vi "Write Results.vi"(8 "error in":errorcluster, 11 "Peer Review in":refnum<class "Peer Review.lvclass">) -> (0 "error out":errorcluster, 3 "Peer Review out":refnum<class "Peer Review.lvclass">)   [LabVIEW 2020, in "Peer Review.lvclass"]
uses:
  Peer Review.lvclass
  Peer Review.lvclass/Peer Review.ctl
  TypeDefs/File Info.ctl
  TypeDefs/File State.ctl
  TypeDefs/VI Type.ctl
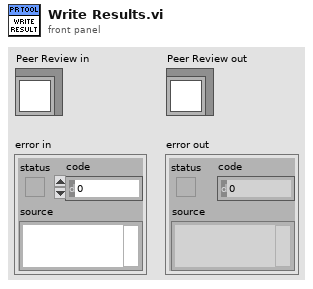
[diagram p1: front panel]
types:
  T1 = typedef "Peer Review.lvclass/File Info.ctl" = cluster{"File ID":i32, "Commit ID":i32, "Reviewed Hash":string, "Relative Path":string, "File Path":path, "File Checksum":string, "State":T2, "FP Changes":i32, "BD Changes":i32, "FP Bounds Error":dbl, "BD Bounds Error":dbl, "Lines Added":i32, "Lines Removed":i32, "Analysis Passes":i32, "Analysis Fails":i32, "Attribute Changes":i32, "Reentrancy Changes":string, "Cyclomatic Complexity":i32, "Node Count":i32, "Revision Number":u32, "LabVIEW Version":string, "Description":string, "Master Path":path, "Master Checksum":string, "VI Type":T3, "LabVIEW File":bool, "Review Complete":bool, "File Ref":refnum<vi>}
  T2 = typedef "Peer Review.lvclass/File State.ctl" = enum16{"Interrogation Needed", "Modified", "Deleted", "Added", "Matches Previous", "No Changes", "Moved"}
  T3 = typedef "Peer Review.lvclass/VI Type.ctl" = enum32{"invalid VI type", "Standard VI", "Control VI", "Global VI", "Polymorphic VI", "Configuration VI", "SubSystem", "Facade VI", "Method VI", "Statechart Diagram VI"}
  T4 = enum16{"open", "replace", "create", "open or create", "replace or create", "replace or create with confirmation"}
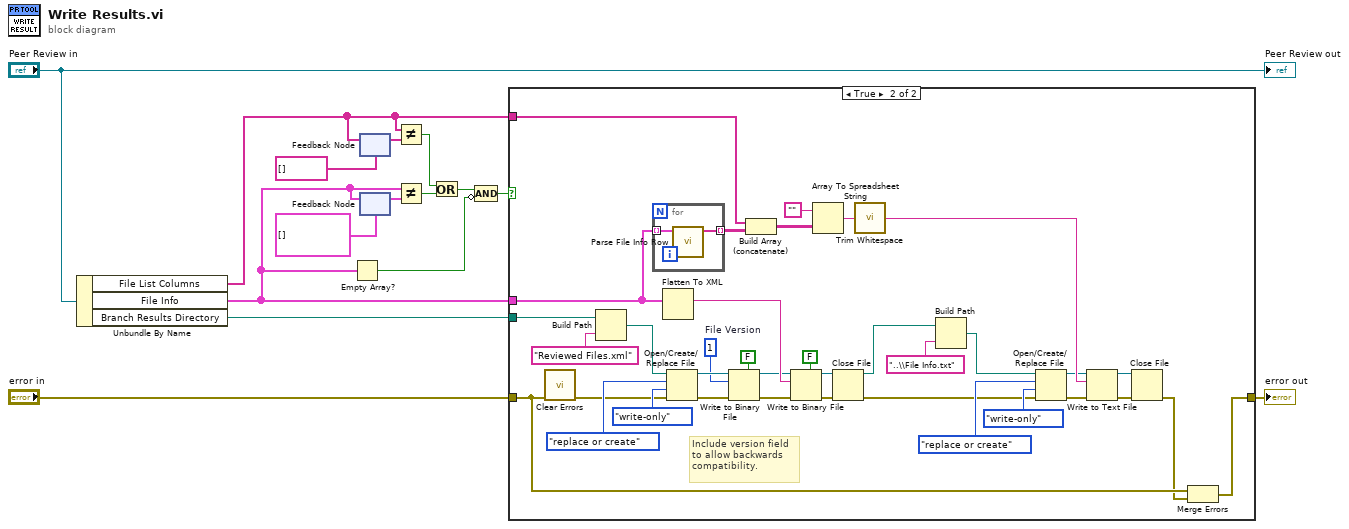
[diagram p0: block diagram]
diagram:
  n1 = Unbundle By Name("Peer Review in") -> ("File List Columns"=w2:string[], "File Info"=w1:T1[], "Branch Results Directory"=w14:path)
  n2 = Empty Array?(array=w1) -> (empty?=w4:bool)
  n3 = feedback #1(string[] [] ("File List Columns")) -> (w10:string[])
  n4 = feedback-in #1(w2) -> ()
  n5 = feedback-in #2(w1) -> ()
  n6 = feedback #2(T1[] [] ("File Info")) -> (w11:T1[])
  n7 = Not Equal?(x=w2, y=w10) -> (x != y?=w9:bool)
  n8 = Not Equal?(x=w1, y=w11) -> (x != y?=w8:bool)
  n9 = Or(x=w9, y=w8) -> (x .or. y?=w5:bool)
  n10 = Compound Arithmetic op=AND(w5, invert w4) -> (w3:bool)
  n11 = case shown="True" w3 {
    tunnel: [w16 w17] -> w12
    tunnel: w14 -> [_ w45]
    tunnel: w1 -> [_ w52]
    tunnel: w2 -> [_ w50]
    tunnel: "error in" -> [w16 w19]
    frame False {
      # "No results to write (or unchanged), so do nothing."
    }
    frame True {
      w33 = u32 1  # File Version
      # "Include version field\nto allow backwards\ncompatibility."
      n12 = call <vilib>:"Clear Errors.vi"("error in (no error)"=w19) -> ("error out"=w20:errorcluster)  [unwired: 5 in, 1 out]
      n13 = Build Path(base path=w45, name or relative path="Reviewed Files.xml") -> (appended path=w39:path)
      n14 = for {
        tunnel: w52 -> [w54] mode=indexing
        tunnel: [w53] -> w51 mode=indexing
        n15 = call "Parse File Info Row.vi"("File Info"=w54) -> ("Column Fields"=w53:string[])  [unwired: 10 in]
      }
      n16 = Flatten To XML(6:w52) -> (2:w38:string)
      n17 = Open/Create/Replace File(file path (use dialog)=w39, error in=w20, operation (0:open)=T4."replace or create", access (0:read/write)=enum16{"read/write", "read-only", "write-only"}."write-only") -> (refnum out=w37:refnum<file>, error out=w35:errorcluster)  [unwired: 2 in, 1 out]
      n18 = Write to Binary File(file (use dialog)=w37, data=w33, error in=w35, 5:FALSE ("prepend array or string size? (T)")) -> (refnum out=w36:refnum<file>, error out=w34:errorcluster)  [unwired: 2 in, 1 out]
      n19 = Build Array (concatenate)(w50, w51) -> (w49:string[][])
      n20 = Write to Binary File(file (use dialog)=w36, data=w38, error in=w34, 5:FALSE ("prepend array or string size? (T)")) -> (refnum out=w42:refnum<file>, error out=w41:errorcluster)  [unwired: 2 in, 1 out]
      n21 = Array To Spreadsheet String(array=w49, 3:"") -> (spreadsheet string=w47:string)  [unwired: 1 in]
      n22 = Close File(refnum=w42, error in=w41) -> (path=w21:path, error out=w23:errorcluster)
      n23 = call <vilib>:"Trim Whitespace.vi"("string"=w47) -> ("trimmed string"=w46:string)  [unwired: 1 in]
      n24 = Build Path(base path=w21, name or relative path="..\\File Info.txt") -> (appended path=w22:path)
      n25 = Open/Create/Replace File(file path (use dialog)=w22, error in=w23, operation (0:open)=T4."replace or create", access (0:read/write)=enum16{"read/write", "read-only", "write-only"}."write-only") -> (refnum out=w27:refnum<file>, error out=w28:errorcluster)  [unwired: 2 in, 1 out]
      n26 = Write to Text File(file (use dialog)=w27, text=w46, error in=w28) -> (refnum out=w29:refnum<file>, error out=w30:errorcluster)  [unwired: 1 in, 1 out]
      n27 = Close File(refnum=w29, error in=w30) -> (error out=w18:errorcluster)  [unwired: 1 out]
      n28 = Merge Errors(w19, w18) -> (w17:errorcluster)
    }
  }
  "error out" <- w12
  "Peer Review out" <- "Peer Review in"
